vi "Enqueue.vi"(8 "error in (no error)":errorcluster, 9 "Data":variant, 10 "Message":string, 11 "Messaging in":refnum<class "Messaging.lvclass">) -> (0 "error out":errorcluster, 3 "Messaging out":refnum<class "Messaging.lvclass">)   [LabVIEW 2023, in "MessagingModule.lvlib" / "Messaging.lvclass"]
uses:
  Messaging.lvclass
  Messaging.lvclass/Messaging.ctl
  Msg/Msg.Data.ctl
  MessagingModule.lvlib
  Msg/Msg.Q.EnqueueMode.ctl
panel:
  in  "Enqueue Mode":T1
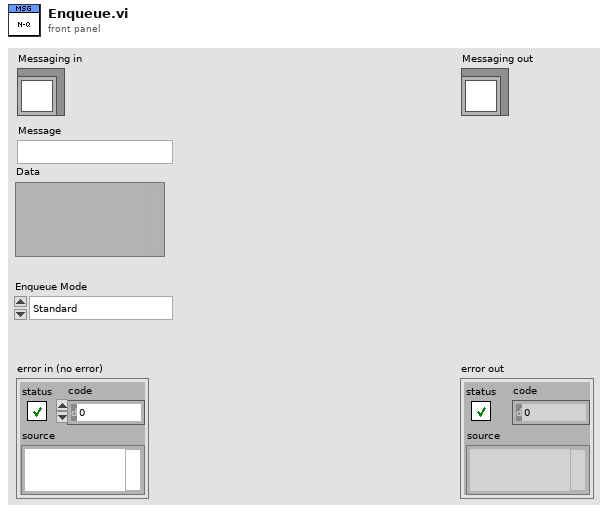
[diagram p1: front panel]
types:
  T1 = typedef "MessagingModule.lvlib/Msg.Q.EnqueueMode.ctl" = enum16{"Standard", "Lossy"}
  T2 = typedef "MessagingModule.lvlib/Msg.Data.ctl" = cluster{"Message":string, "Data":variant}
  T3 = typedef "MessagingModule.lvlib/Msg.Q.Ref.ctl" = refnum<queue>
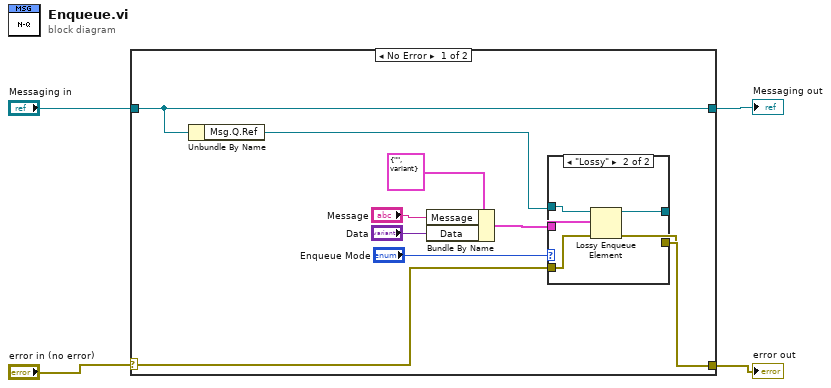
[diagram p0: block diagram]
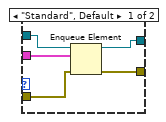
[diagram p2: hidden frame]
diagram:
  n1 = case shown="No Error" "error in (no error)" {
    selector: "error in (no error)" -> [w5 w25]
    tunnel: [w6 w25] -> w3
    tunnel: [w10 w24] -> w1
    tunnel: "Messaging in" -> [w10 w24]
    frame No Error {
      n2 = Unbundle By Name(w10) -> ("Msg.Q.Ref"=w7:T3)
      n3 = Bundle By Name(cluster=T2 {"Message"="", "Data"=variant} ("Msg.Q.Data"), "Message"="Message", "Data"="Data") -> (w9:T2)
      n4 = case shown="\"Lossy\"" "Enqueue Mode" {
        tunnel: w7 -> [w15 w19]
        tunnel: [w18 w21] -> _
        tunnel: [w17 w22] -> w6
        tunnel: w9 -> [w16 w23]
        tunnel: w5 -> [w14 w20]
        frame "Standard", Default {
          n5 = Enqueue Element(queue=w15, element=w16, error in (no error)=w14) -> (queue out=w18:T3, error out=w17:errorcluster)  [unwired: 1 in, 1 out]
        }
        frame "Lossy" {
          n6 = Lossy Enqueue Element(queue=w19, element=w23, error in (no error)=w20) -> (queue out=w21:T3, error out=w22:errorcluster)  [unwired: 2 out]
        }
      }
    }
    frame Error {
    }
  }
  "error out" <- w3
  "Messaging out" <- w1
